vi "String Subset.vi"(8 "error in (no error)":errorcluster, 9 "Length in Bytes (0)":i32, 10 "Byte Offset (0)":i32, 11 "UTF8 in":refnum<class "UTF-8 String.lvclass">) -> (0 "error out":errorcluster, 2 "String Subset":string, 3 "UTF8 out":refnum<class "UTF-8 String.lvclass">)   [LabVIEW 2019, in "JKI Unicode.lvlib" / "UTF-8 String.lvclass"]
doc: "JKI Unicode 1.0.0.7\nTomi Maila - JKI\nCopyright (c) 2016, JKI"
uses:
  UTF-8 String.lvclass
  UTF-8 String.lvclass/UTF-8 String.ctl
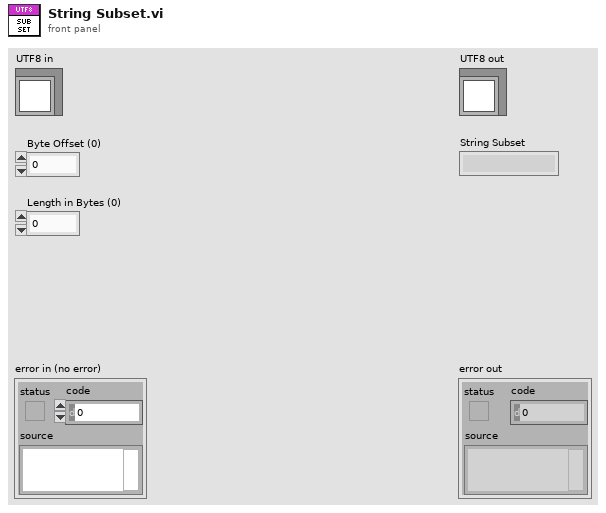
[diagram p1: front panel]
types:
  T1 = typedef "JKI Unicode.lvlib/UTF-8 String.lvclass/Byte Stream.ctl" = u8[]
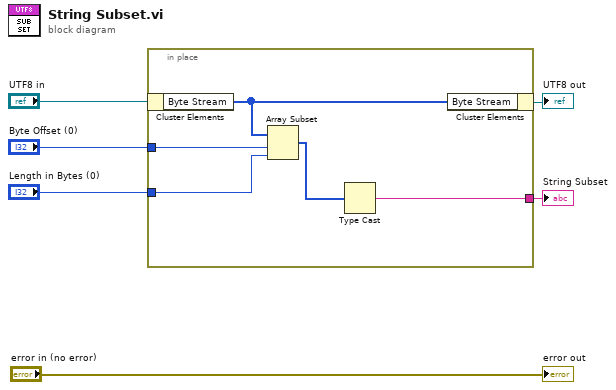
[diagram p0: block diagram]
diagram:
  n1 = in-place {
    in-place-border: "Byte Offset (0)" -> [w11]
    in-place-border: "Length in Bytes (0)" -> [w10]
    in-place-border: [w7] -> w1
    n2 = in-place-cluster #1("UTF8 in") -> ("Byte Stream"=w9:T1)
    n3 = Array Subset(array=w9, index=w11, length=w10) -> (w8:T1)
    n4 = Type Cast(x=w8) -> (*(type *) &x=w7:string)  [unwired: 1 in]
    n5 = in-place-cluster #1("Byte Stream"=w9) -> (→"UTF8 out":refnum<class "UTF-8 String.lvclass">)
  }
  "String Subset" <- w1
  "error out" <- "error in (no error)"
